vi "Writie Timing Src Properties.vi"(8 "Error In":errorcluster, 10 "Timing Source Properties":T1, 11 "Custom Device .NET Ref In":refnum<k24>) -> (0 "Error Out":errorcluster, 3 "Custom Device .NET Ref Out":refnum<k24>)   [LabVIEW 2019, in "VeriStand Custom Device XML Parser.lvlib"]
doc: "If the custom device is a timing source, this writes the properties of that source to the custom device."
uses:
  VeriStand Custom Device XML Parser.lvlib
  NationalInstruments.VeriStand.XMLReader
  XML Controls/Timing Source Properties.ctl
  XML Controls/Timing Source Source Distribution Properties.ctl
  XML Controls/Supported Targets.ctl
  XML Controls/Path Cluster.ctl
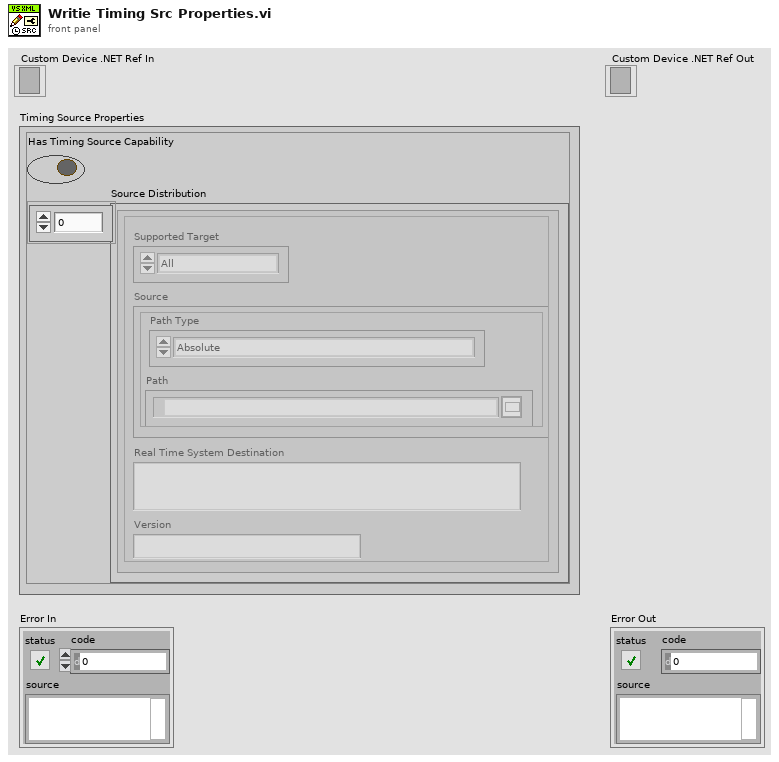
[diagram p1: front panel]
types:
  T1 = typedef "VeriStand Custom Device XML Parser.lvlib/Timing Source Properties.ctl" = cluster{"Has Timing Source Capability":bool, "Source Distribution":T2}
  T2 = typedef "VeriStand Custom Device XML Parser.lvlib/Timing Source Source Distribution Properties.ctl" = cluster{"Supported Target":T3, "Source":T4, "Real Time System Destination":string, "Version":string}[]
  T3 = typedef "VeriStand Custom Device XML Parser.lvlib/Supported Targets.ctl" = enum16{"All", "Pharlap", "VxWorks", "Windows", "Linux_32_ARM", "Linux_x64", "PharlapWindows", "PharlapVxWorks", "VxWorksWindows"}
  T4 = typedef "VeriStand Custom Device XML Parser.lvlib/Path Cluster.ctl" = cluster{"Path":path, "Path Type":enum16{"Absolute", "To Base", "To Common Doc Dir", "To Application Data Dir"}}
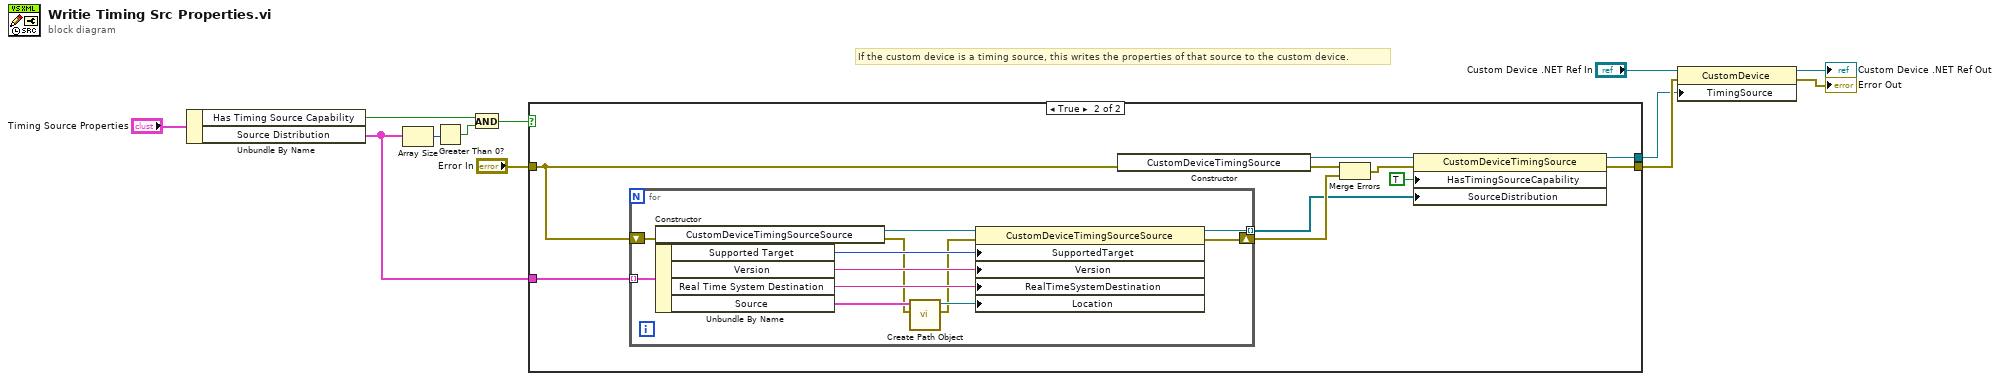
[diagram p0: block diagram]
diagram:
  # "If the custom device is a timing source, this writes the properties of that source to the custom device."
  n1 = Unbundle By Name("Timing Source Properties") -> ("Has Timing Source Capability"=w5:bool, "Source Distribution"=w8:T2)
  n2 = Array Size(array=w8) -> (size(s)=w3:i32)
  n3 = Greater Than 0?(x=w3) -> (x > 0?=w4:bool)
  n4 = And(x=w5, y=w4) -> (x .and. y?=w6:bool)
  n5 = case shown="True" w6 {
    tunnel: "Error In" -> [w13 w21]
    tunnel: w8 -> [_ w20]
    tunnel: [_ w15] -> w9
    tunnel: [w13 w14] -> w10
    frame False {
    }
    frame True {
      n6 = for {
        shift-right: [w29] -> w17
        shift-left: w21 -> [w30]
        tunnel: w20 -> [w34] mode=indexing
        tunnel: [w28] -> w16 mode=indexing
        n7 = constructor class="CustomDeviceTimingSourceSource"(error in=w30) -> (reference out=w35:refnum<k24>, error out=w26:errorcluster)  [unwired: 2 in, 1 out]
        n8 = Unbundle By Name(w34) -> ("Supported Target"=w33:T3, "Version"=w32:string, "Real Time System Destination"=w31:string, "Source"=w27:T4)
        n9 = call "Create Path Object.vi"("Error In"=w26, "Path Data Cluster"=w27) -> ("Error Out"=w24:errorcluster, "Path .NET Ref"=w25:refnum<k24>)  [unwired: 8 in]
        n10 = property class="CustomDeviceTimingSourceSource"(reference=w35, error in=w24, "SupportedTarget"=w33, "Version"=w32, "RealTimeSystemDestination"=w31, "Location"=w25) -> (reference out=w28:refnum<k24>, error out=w29:errorcluster)
      }
      n11 = constructor class="CustomDeviceTimingSource"(error in=w21) -> (reference out=w23:refnum<k24>, error out=w19:errorcluster)  [unwired: 2 in, 1 out]
      n12 = Merge Errors(w19, w17) -> (w18:errorcluster)
      n13 = property class="CustomDeviceTimingSource"(reference=w23, error in=w18, "HasTimingSourceCapability"=TRUE, "SourceDistribution"=w16) -> (reference out=w15:refnum<k24>, error out=w14:errorcluster)
    }
  }
  n14 = property class="CustomDevice"(reference="Custom Device .NET Ref In", error in=w10, "TimingSource"=w9) -> (reference out=→"Custom Device .NET Ref Out":refnum<k24>, error out=→"Error Out":errorcluster)
